vi "Write Data Value Refs.vi"(8 "error in (no error)":errorcluster, 10 "Type Counts":T1, 11 "Local Bus in":refnum<class "Local Bus.lvclass">) -> (0 "error out":errorcluster, 3 "Local Bus out":refnum<class "Local Bus.lvclass">)   [LabVIEW 2021, in "Local Bus.lvclass"]
uses:
  Local Bus.lvclass
  Local Bus.lvclass/Local Bus.ctl
  Support/Data Value References.ctl
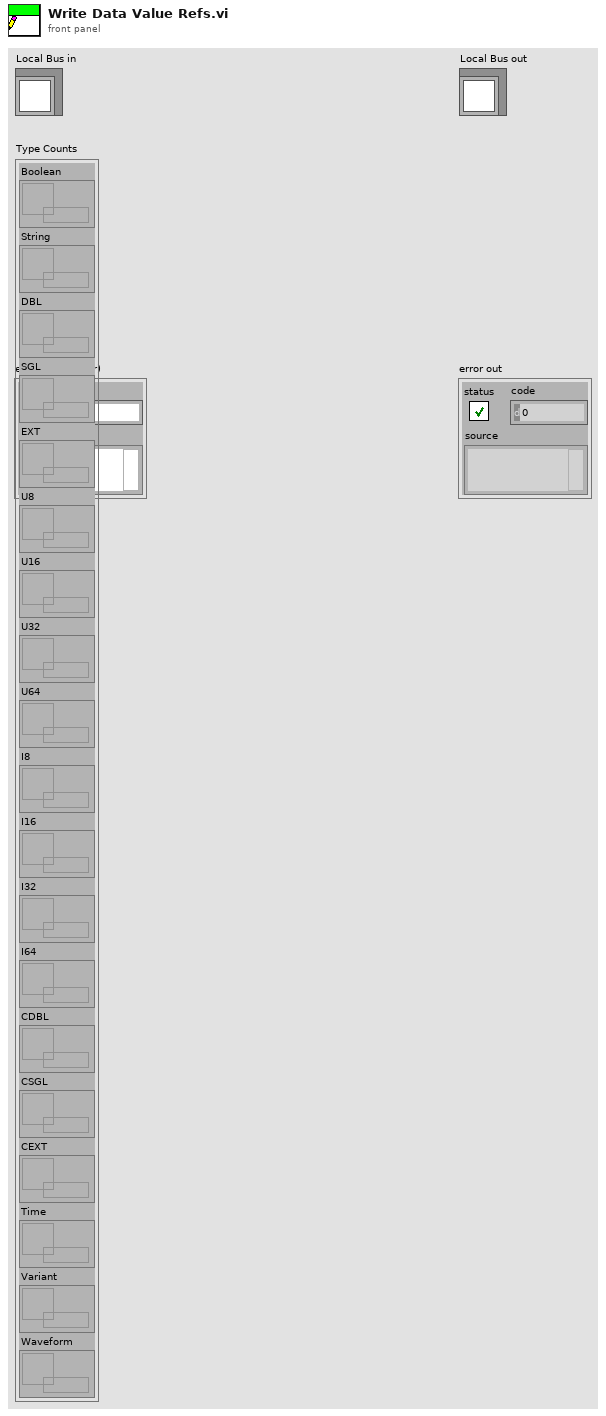
[diagram p1: front panel]
types:
  T1 = typedef "Local Bus.lvclass/Data Value References.ctl" = cluster{"Boolean":refnum<data-value>, "String":refnum<data-value>, "DBL":refnum<data-value>, "SGL":refnum<data-value>, "EXT":refnum<data-value>, "U8":refnum<data-value>, "U16":refnum<data-value>, "U32":refnum<data-value>, "U64":refnum<data-value>, "I8":refnum<data-value>, "I16":refnum<data-value>, "I32":refnum<data-value>, "I64":refnum<data-value>, "CDBL":refnum<data-value>, "CSGL":refnum<data-value>, "CEXT":refnum<data-value>, "Time":refnum<data-value>, "Variant":refnum<data-value>, "Waveform":refnum<data-value>}
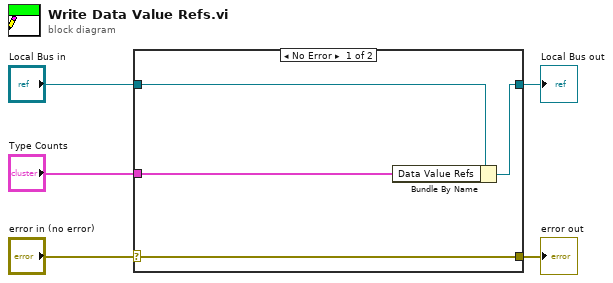
[diagram p0: block diagram]
diagram:
  n1 = case shown="No Error" "error in (no error)" {
    selector: "error in (no error)" -> [w9 w10]
    tunnel: [w9 w10] -> w4
    tunnel: [w7 w11] -> w2
    tunnel: "Local Bus in" -> [w8 w11]
    tunnel: "Type Counts" -> [w6 _]
    frame No Error {
      n2 = Bundle By Name(cluster=w8, "Data Value Refs"=w6) -> (w7:refnum<class "Local Bus.lvclass">)
    }
    frame Error {
    }
  }
  "error out" <- w4
  "Local Bus out" <- w2
